vi "Calculate Exponential Fuel Cost.vi"(11 "Numeric":i32) -> (3 "Numeric 2":i32)   [LabVIEW 2019, in "Day 7.lvlib"]
uses:
  Day 7.lvlib
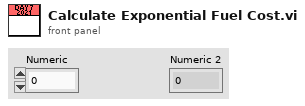
[diagram p1: front panel]
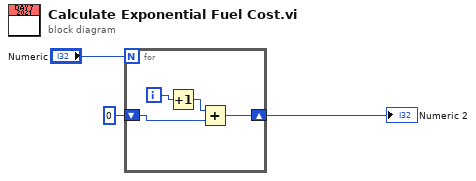
[diagram p0: block diagram]
diagram:
  n1 = for {
    N: "Numeric" -> [_]
    shift-right: [w7] -> w1
    shift-left: 0 -> [w6]
    i -> [w5]
    n2 = Increment(x=w5) -> (x+1=w4:i32)
    n3 = Add(x=w4, y=w6) -> (x+y=w7:i32)
  }
  "Numeric 2" <- w1
